vi "Text to Graphic Font.vi"(11 "Text Font":T2) -> (3 "Graphic Font":T1)   [LabVIEW 2015, in "BreadcrumbNavigator.lvclass"]
uses:
  BreadcrumbNavigator.lvclass
  <vilib>/Utility/miscctls.llb/LVFontTypeDef.ctl
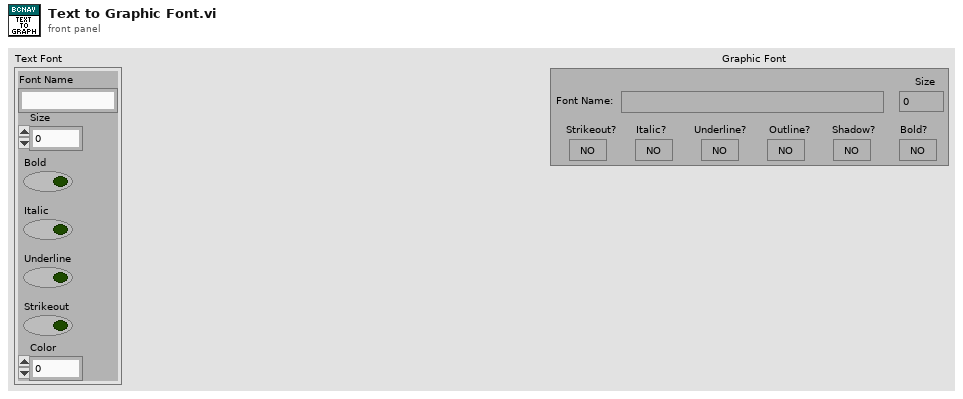
[diagram p1: front panel]
types:
  T1 = cluster{"Font Name:":string, "Size":i16, "Strikeout?":bool, "Italic?":bool, "Underline?":bool, "Outline?":bool, "Shadow?":bool, "Bold?":bool}
  T2 = typedef "LVFontTypeDef.ctl" = cluster{"Font Name":string, "Size":u16, "Bold":bool, "Italic":bool, "Underline":bool, "Strikeout":bool, "Color":u32}
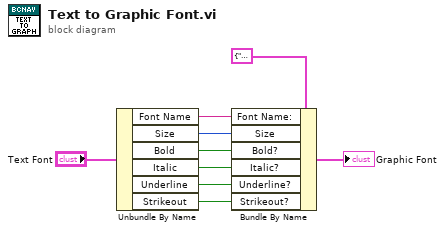
[diagram p0: block diagram]
diagram:
  n1 = Unbundle By Name("Text Font") -> ("Font Name"=w7:string, "Size"=w6:u16, "Bold"=w5:bool, "Italic"=w4:bool, "Underline"=w3:bool, "Strikeout"=w2:bool)
  n2 = Bundle By Name(cluster=T1 {"Font Name:"="", "Size"=0, "Strikeout?"=FALSE, "Italic?"=FALSE, "Underline?"=FALSE, "Outline?"=FALSE, "Shadow?"=FALSE, "Bold?"=FALSE} ("Graphic Font"), "Font Name:"=w7, "Size"=w6, "Bold?"=w5, "Italic?"=w4, "Underline?"=w3, "Strikeout?"=w2) -> (→"Graphic Font":T1)
